vi "parse_CMDState.vi"(8 "error in":errorcluster, 11 "msg in":string) -> (0 "error out":errorcluster, 2 "CMD State":T1, 3 "msg out":string)   [LabVIEW 2018]
uses:
  <userlib>/ROS for LabVIEW Software/ROS/MessageParsing/std_msgs/subs/parse_float64_scalar.vi
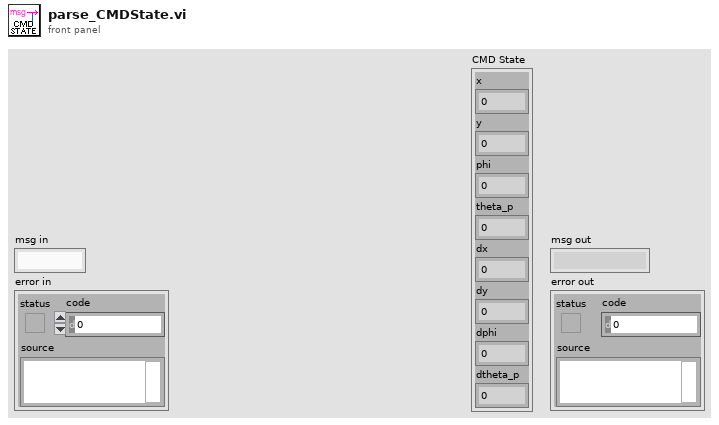
[diagram p1: front panel]
types:
  T1 = cluster{"x":dbl, "y":dbl, "phi":dbl, "theta_p":dbl, "dx":dbl, "dy":dbl, "dphi":dbl, "dtheta_p":dbl}
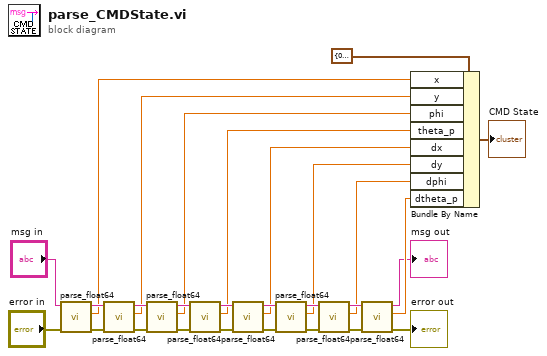
[diagram p0: block diagram]
diagram:
  n1 = call-poly <userlib>:"parse_float64.vi"("error in"="error in", "msg in"="msg in") -> ("error out"=w18:errorcluster, "number"=w10:dbl, "msg out"=w26:string)  [unwired: 3 in]
  n2 = call-poly <userlib>:"parse_float64.vi"("error in"=w18, "msg in"=w26) -> ("error out"=w17:errorcluster, "number"=w9:dbl, "msg out"=w25:string)  [unwired: 3 in]
  n3 = call-poly <userlib>:"parse_float64.vi"("error in"=w17, "msg in"=w25) -> ("error out"=w16:errorcluster, "number"=w8:dbl, "msg out"=w24:string)  [unwired: 3 in]
  n4 = call-poly <userlib>:"parse_float64.vi"("error in"=w16, "msg in"=w24) -> ("error out"=w15:errorcluster, "number"=w7:dbl, "msg out"=w23:string)  [unwired: 3 in]
  n5 = call-poly <userlib>:"parse_float64.vi"("error in"=w15, "msg in"=w23) -> ("error out"=w14:errorcluster, "number"=w6:dbl, "msg out"=w22:string)  [unwired: 3 in]
  n6 = call-poly <userlib>:"parse_float64.vi"("error in"=w14, "msg in"=w22) -> ("error out"=w13:errorcluster, "number"=w5:dbl, "msg out"=w21:string)  [unwired: 3 in]
  n7 = call-poly <userlib>:"parse_float64.vi"("error in"=w13, "msg in"=w21) -> ("error out"=w12:errorcluster, "number"=w4:dbl, "msg out"=w20:string)  [unwired: 3 in]
  n8 = call-poly <userlib>:"parse_float64.vi"("error in"=w12, "msg in"=w20) -> ("error out"=→"error out":errorcluster, "number"=w3:dbl, "msg out"=→"msg out":string)  [unwired: 3 in]
  n9 = Bundle By Name(cluster=T1 {"x"=0.0, "y"=0.0, "phi"=0.0, "theta_p"=0.0, "dx"=0.0, "dy"=0.0, "dphi"=0.0, "dtheta_p"=0.0} ("State"), "x"=w10, "y"=w9, "phi"=w8, "theta_p"=w7, "dx"=w6, "dy"=w5, "dphi"=w4, "dtheta_p"=w3) -> (→"CMD State":T1)
